vi "sensoreshumedad.vi"() -> ()   [LabVIEW 2020]
panel:
  out "Datos":string="Humedad_sulo_1"
  out "Datos":string="Humedad_sulo_1"
  in  "address":string
  in  "remote port":u16
  out "Voltaje 3":i32
  out "Voltaje 2":dbl(slide) scale=0.0..5.0
  out "Waveform Chart 2":dbl(graph)
  out "Voltaje":dbl(slide) scale=0.0..5.0
  out "Waveform Chart":dbl(graph)
  out "Voltaje":i32
  in  "stop":bool
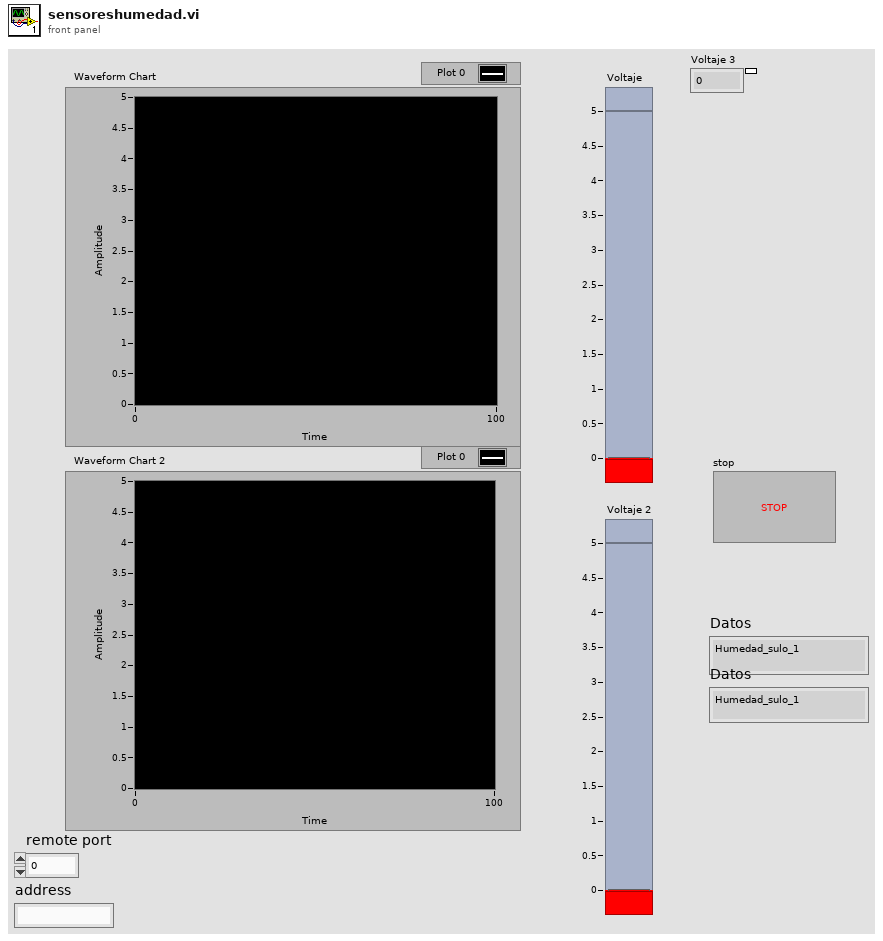
[diagram p1: front panel]
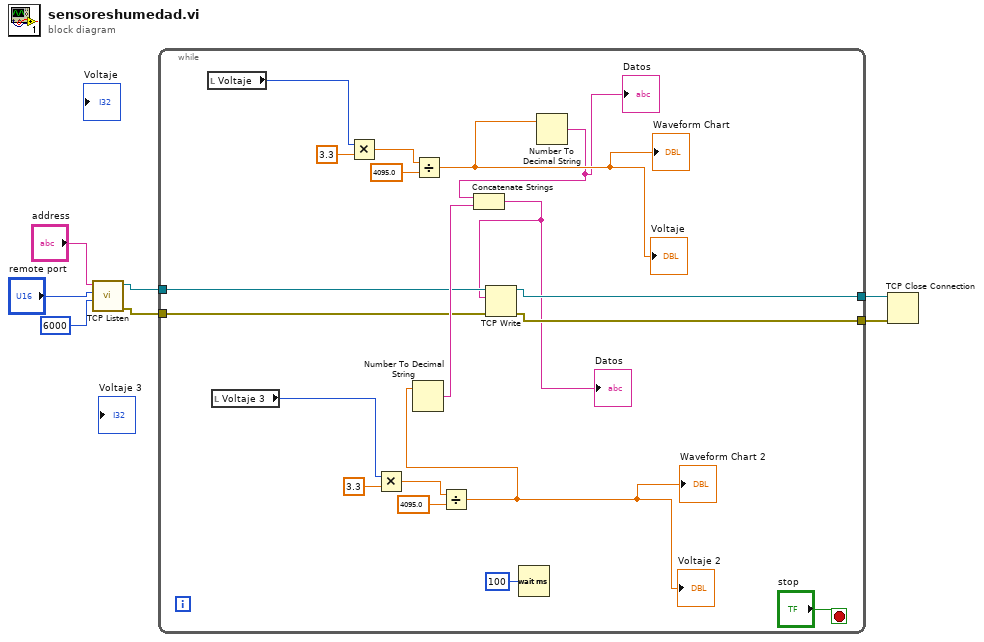
[diagram p0: block diagram]
diagram:
  n1 = call <vilib>:"TCP Listen.vi"("timeout ms (wait forever: -1)"=6000 ("timeout ms (60000)"), "port"="remote port", "service name"="address") -> ("error out"=w4:errorcluster, "connection ID"=w5:refnum<k5>)  [unwired: 4 in, 3 out]
  n2 = while {
    tunnel: [w10] -> w7
    tunnel: [w12] -> w6
    tunnel: w5 -> [w13]
    tunnel: w4 -> [w11]
    stop <- "stop" stop-if-true
    n3 = local read "Voltaje"() -> (w23:i32)
    n4 = local read "Voltaje 3"() -> (w17:i32)
    n5 = Multiply(x=w23, y=3.3) -> (x*y=w22:dbl)
    n6 = Multiply(x=w17, y=3.3) -> (x*y=w20:dbl)
    n7 = Divide(x=w22, y=4095.0) -> (x/y=w15:dbl)
    "Waveform Chart" <- w15
    "Voltaje" <- w15
    n8 = Divide(x=w20, y=4095.0) -> (x/y=w14:dbl)
    "Waveform Chart 2" <- w14
    "Voltaje 2" <- w14
    n9 = Number To Decimal String(number=w14) -> (decimal integer string=w16:string)  [unwired: 1 in]
    n10 = Wait (ms)(milliseconds to wait=u32 100) -> ()  [unwired: 1 out]
    n11 = Number To Decimal String(number=w15) -> (decimal integer string=w9:string)  [unwired: 1 in]
    "Datos" <- w9
    n12 = Concatenate Strings(w9, w16) -> (w8:string)
    "Datos" <- w8
    n13 = TCP Write(connection ID=w13, data in=w8, error in (no error)=w11) -> (connection ID out=w12:refnum<k5>, error out=w10:errorcluster)  [unwired: 1 in, 1 out]
  }
  n14 = TCP Close Connection(connection ID=w6, error in (no error)=w7) -> ()  [unwired: 1 in, 2 out]
